vi "Teardown.vi"(8 "error in":errorcluster, 11 "_Rescript in":refnum<class "_Rescript.lvclass">) -> (0 "error out":errorcluster)   [LabVIEW 2020, in "_Rescript.lvlib" / "_Rescript.lvclass"]
uses:
  _Rescript.lvclass
  _Rescript.lvclass/_Rescript.ctl
  _Shared/Project Stuff/Project Stuff.lvclass
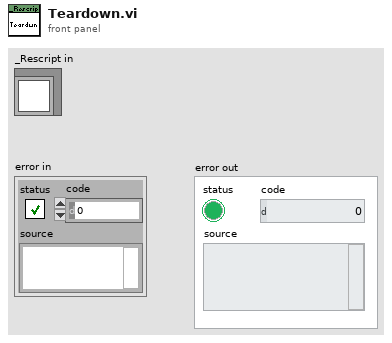
[diagram p1: front panel]
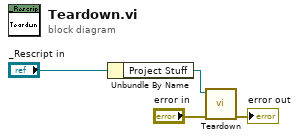
[diagram p0: block diagram]
diagram:
  n1 = Unbundle By Name("_Rescript in") -> ("Project Stuff"=w3:refnum<class "Project Stuff.lvclass">)
  n2 = call "Teardown.vi"("Error in"="error in", "Project Stuff in"=w3) -> ("Error out"=→"error out":errorcluster)  [unwired: 9 in]
